vi "wrapWithConditionalDisableStructure.vi"(6 "Node Refnum CDS Source":refnum<vi>, 8 "error in (no error)":errorcluster, 9 "Block Diagram":refnum<vi>, 10 "Node Refnum CLFN":refnum<vi>, 11 "VI in":refnum<class "VI.lvclass">) -> (0 "error out":errorcluster, 2 "Node Refnum CDS New":refnum<vi>, 3 "VI out":refnum<class "VI.lvclass">)   [LabVIEW 2016, in "VI.lvclass"]
uses:
  VI.lvclass
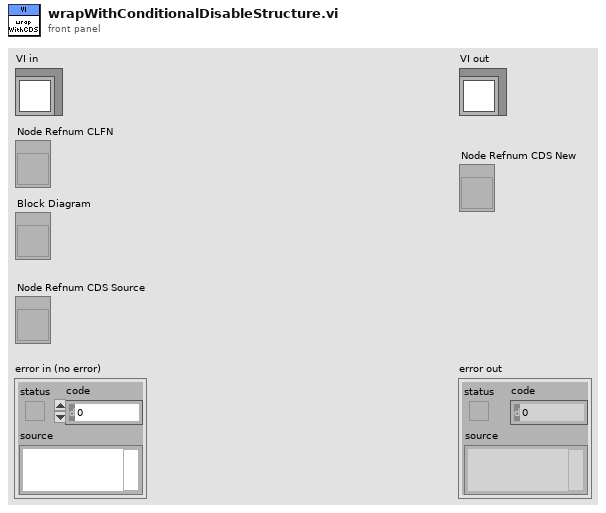
[diagram p1: front panel]
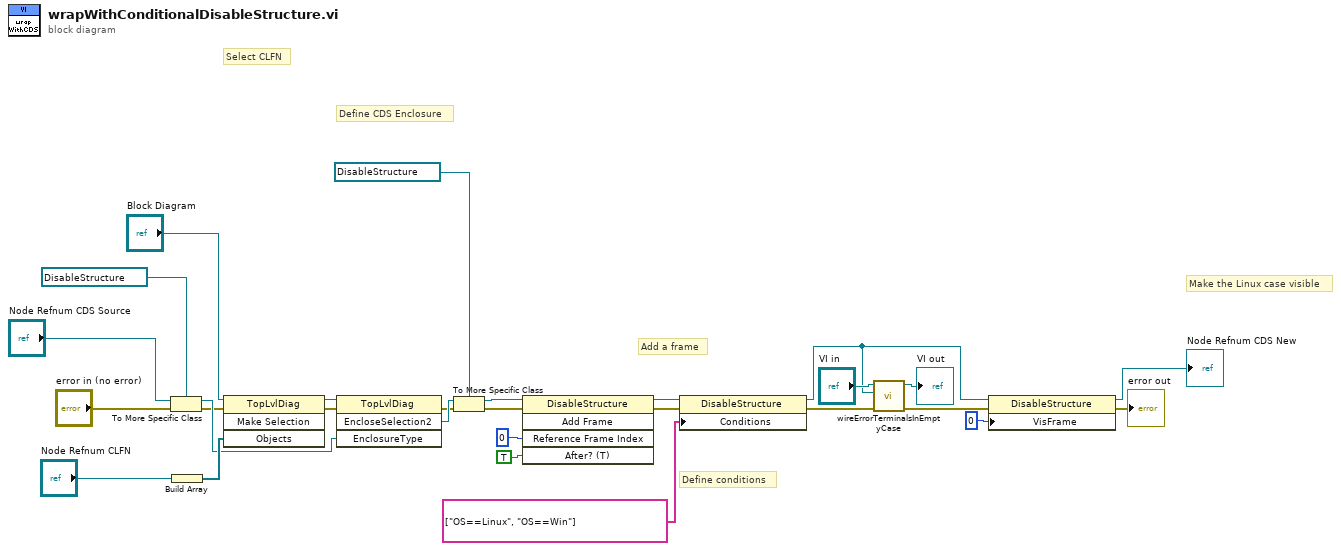
[diagram p0: block diagram]
diagram:
  # "Make the Linux case visible"
  # "Define conditions"
  # "Add a frame"
  # "Define CDS Enclosure"
  # "Select CLFN"
  n1 = To More Specific Class(target class=refnum<vi> refnum ("EnclosureType"), reference="Node Refnum CDS Source", error in="error in (no error)") -> (specific class reference=w24:refnum<vi>, error out=w11:errorcluster)
  n2 = Build Array("Node Refnum CLFN") -> (w28:refnum<vi>[])
  n3 = invoke class="TopLvlDiag" method="Make Selection"(reference="Block Diagram", error in=w11, "Objects"=w28) -> (reference out=w27:refnum<vi>, error out=w26:errorcluster)  [unwired: 1 in, 2 out]
  n4 = invoke class="TopLvlDiag" method="EncloseSelection2"(reference=w27, error in=w26, "EnclosureType"=w24) -> (error out=w10:errorcluster, "EncloseSelection2"=w22:refnum<vi>)  [unwired: 1 in, 2 out]
  n5 = To More Specific Class(target class=refnum<vi> refnum ("EnclosureType"), reference=w22, error in=w10) -> (specific class reference=w21:refnum<vi>, error out=w9:errorcluster)
  n6 = invoke class="DisableStructure" method="Add Frame"(reference=w21, error in=w9, "Reference Frame Index"=u32 0, "After? (T)"=TRUE) -> (reference out=w20:refnum<vi>, error out=w8:errorcluster)  [unwired: 1 in, 3 out]
  n7 = property class="DisableStructure"(reference=w20, error in=w8, "Conditions"=string[] ["OS==Linux", "OS==Win"]) -> (reference out=w2:refnum<vi>, error out=w4:errorcluster)
  n8 = call "wireErrorTerminalsInEmptyCase.vi"("error in (no error)"=w4, "reference out_CDSNew"=w2, "VI in"="VI in") -> ("error out"=w3:errorcluster, "VI out"=→"VI out":refnum<class "VI.lvclass">)  [unwired: 7 in]
  n9 = property class="DisableStructure"(reference=w2, error in=w3, "VisFrame"=u32 0 ("Visible Frame")) -> (reference out=→"Node Refnum CDS New":refnum<vi>, error out=→"error out":errorcluster)
